vi "Configure List Step Parameter.vi"(6 "Step Time(1)":dbl=1.0, 8 "error in (no error)":errorcluster, 9 "List Step Number(2)":dbl=2.0, 10 "Unit(S)":u16(ring) items=["S", "mS"], 11 "VISA resource name":refnum<visa-resource-name>) -> (0 "error out":errorcluster, 3 "VISA resource name out":refnum<visa-resource-name>)   [LabVIEW 2021, in "Keithley 2200 Series.lvlib"]
doc: "Sets the value for the parameter of one list step,indicated by List step number,Step time and units for the list width in either seconds (SECOND) or milliseconds (MSECOND). ."
uses:
  <instrlib>/Keithley 2200 Series/Keithley 2200 Series.lvlib
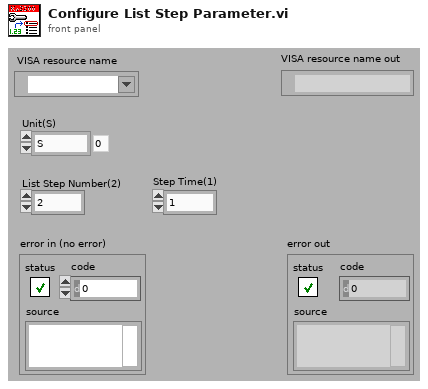
[diagram p1: front panel]
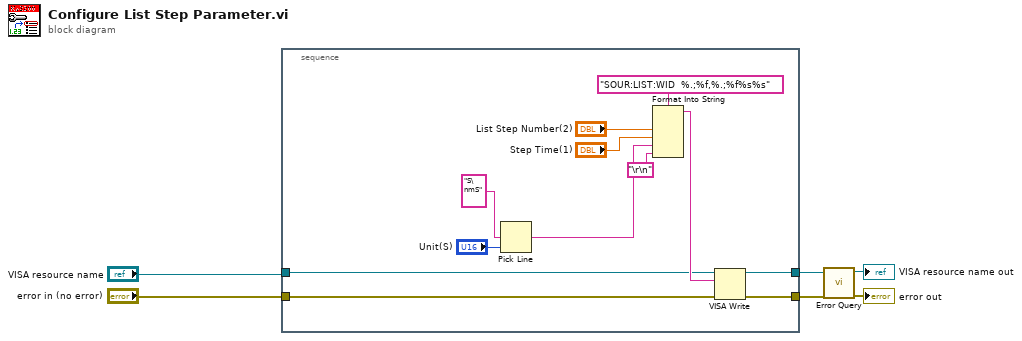
[diagram p0: block diagram]
diagram:
  n1 = stacked-sequence {
    tunnel: [w18] -> w6
    tunnel: [w17] -> w5
    tunnel: "VISA resource name" -> [w13]
    tunnel: "error in (no error)" -> [w12]
    frame #0 {
      n2 = Pick Line(multi-line string="S\nmS", line index="Unit(S)") -> (output string=w7:string)  [unwired: 1 out]
      n3 = Format Into String(format string="SOUR:LIST:WID  %.;%f,%.;%f%s%s", "List Step Number(2)", "Step Time(1)", w7, "\r\n") -> (resulting string=w15:string)  [unwired: 2 in, 1 out]
      n4 = VISA Write(VISA resource name=w13, write buffer=w15, error in (no error)=w12) -> (VISA resource name out=w18:refnum<visa-resource-name>, error out=w17:errorcluster)  [unwired: 1 out]
    }
  }
  n5 = call <instrlib>:"Error Query.vi"("error in (no error)"=w5, "VISA resource name"=w6) -> ("error out"=→"error out":errorcluster, "VISA resource name out"=→"VISA resource name out":refnum<visa-resource-name>)  [unwired: 8 out]
